vi "dfd_Get Stopband Matrix (Odd).vi"(7 "number of bands":i32=4, 9 "roll off":dbl, 11 "order":i32) -> (2 "Us":dbl[][](array[numeric]))   [LabVIEW 2017, in "NI_DigFilter_FilterBank.lvlib"]
uses:
  <vilib>/addons/Digital Filter Design/NI_DigFilter_FilterBank.lvlib
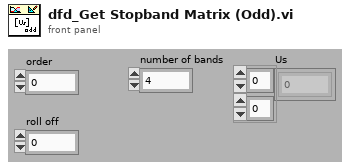
[diagram p1: front panel]
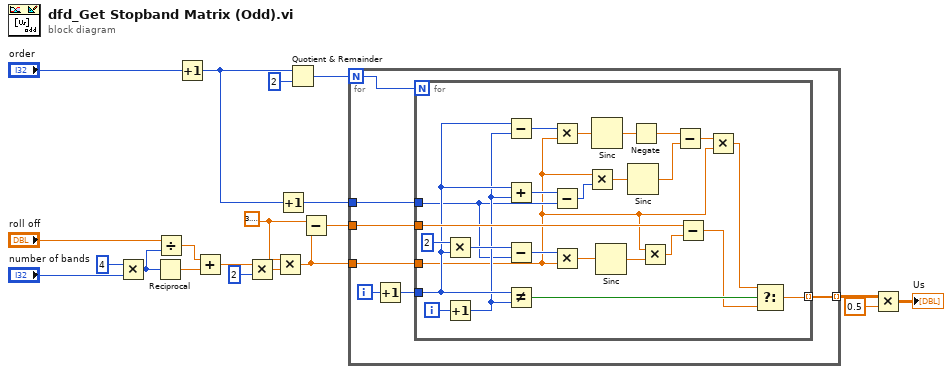
[diagram p0: block diagram]
diagram:
  w20 = 3.141592653589793
  n1 = Multiply(x=4, y="number of bands") -> (x*y=w8:i32)
  n2 = Reciprocal(x=w8) -> (1/x=w1:dbl)
  n3 = Divide(x="roll off", y=w8) -> (x/y=w2:dbl)
  n4 = Increment(x="order") -> (x+1=w7:i32)
  n5 = Add(x=w2, y=w1) -> (x+y=w13:dbl)
  n6 = Multiply(x=w13, y=2) -> (x*y=w11:dbl)
  n7 = Multiply(x=w20, y=w11) -> (x*y=w15:dbl)
  n8 = Increment(x=w7) -> (x+1=w16:i32)
  n9 = Quotient & Remainder(x=w7, y=2) -> (floor(x/y)=w17:i32)  [unwired: 1 out]
  n10 = Subtract(x=w20, y=w15) -> (x-y=w18:dbl)
  n11 = for {
    N: w17 -> [w26]
    tunnel: w16 -> [w24]
    tunnel: w15 -> [w23]
    tunnel: w18 -> [w22]
    tunnel: [w21] -> w5 mode=indexing
    i -> [w27]
    n12 = Increment(x=w27) -> (x+1=w25:i32)
    n13 = for {
      N: w26 -> [_]
      tunnel: w25 -> [w43]
      tunnel: w24 -> [w40]
      tunnel: w23 -> [w30]
      tunnel: w22 -> [w46]
      tunnel: [w37] -> w21 mode=indexing
      i -> [w52]
      n14 = Multiply(x=2, y=w43) -> (x*y=w50:i32)
      n15 = Increment(x=w52) -> (x+1=w42:i32)
      n16 = Subtract(x=w43, y=w42) -> (x-y=w36:i32)
      n17 = Add(x=w43, y=w42) -> (x+y=w41:i32)
      n18 = Subtract(x=w50, y=w40) -> (x-y=w48:i32)
      n19 = Not Equal?(x=w43, y=w42) -> (x != y?=w45:bool)
      n20 = Multiply(x=w36, y=w30) -> (x*y=w44:dbl)
      n21 = Subtract(x=w41, y=w40) -> (x-y=w38:i32)
      n22 = Multiply(x=w48, y=w30) -> (x*y=w49:dbl)
      n23 = Multiply(x=w30, y=w38) -> (x*y=w39:dbl)
      n24 = Sinc(1:w44) -> (0:w32:dbl)
      n25 = Sinc(1:w49) -> (0:w34:dbl)
      n26 = Sinc(1:w39) -> (0:w33:dbl)
      n27 = Negate(x=w32) -> (-x=w35:dbl)
      n28 = Multiply(x=w30, y=w34) -> (x*y=w47:dbl)
      n29 = Subtract(x=w35, y=w33) -> (x-y=w31:dbl)
      n30 = Subtract(x=w46, y=w47) -> (x-y=w28:dbl)
      n31 = Multiply(x=w31, y=w30) -> (x*y=w29:dbl)
      n32 = Select(t=w29, s=w45, f=w28) -> (s? t:f=w37:dbl)
    }
  }
  n33 = Multiply(x=w5, y=0.5) -> (x*y=→"Us":dbl[][])
